vi "Clusters.vi"() -> ()   [LabVIEW 2020]
panel:
  out "cluster 2":T1
  out "cluster":T2
  in  "Array 2":dbl[](array[knob]) scale=0.0..10.0
  out "array":bool[](array[boolean])
  in  "Cluster":T3
  out "output cluster 2":T4
  in  "Array":bool[](array[boolean])
  in  "Tank":i16(slide) scale=0.0..10.0
  in  "String":string
  in  "Horizontal Pointer Slide":dbl(slide) scale=0.0..10.0
  out "output cluster":T5
  out "RPM 2":dbl
  in  "Knob":dbl(knob) scale=0.0..10.0
  out "Stop Button":bool
  out "RPM":dbl
  out "Motor1":bool
  out "Send Data":string
  out "Termocupla":dbl
  in  "Cluster1":T5 {"RPM" scale=0.0..10.0; "Termocupla" scale=0.0..100.0}
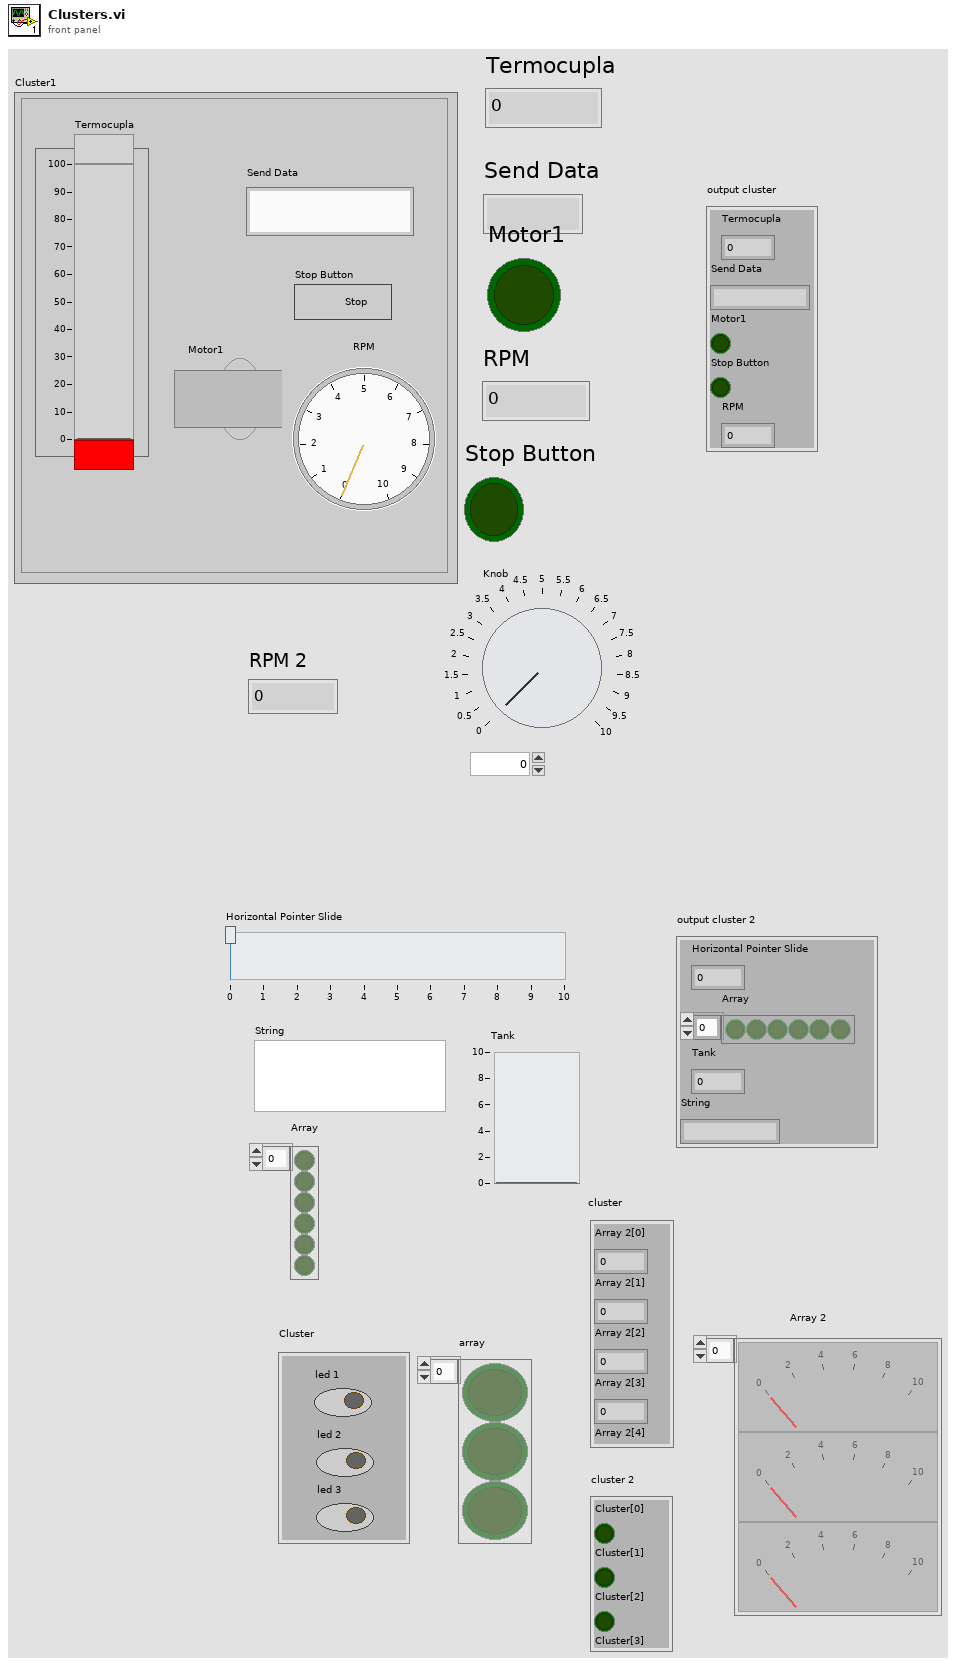
[diagram p1: front panel]
types:
  T1 = cluster{"Cluster[0]":bool, "Cluster[1]":bool, "Cluster[2]":bool, "Cluster[3]":bool, "Cluster[4]":bool, "Cluster[5]":bool, "Cluster[6]":bool, "Cluster[7]":bool, "Cluster[8]":bool}
  T2 = cluster{"Array 2[0]":dbl, "Array 2[1]":dbl, "Array 2[2]":dbl, "Array 2[3]":dbl, "Array 2[4]":dbl, "Array 2[5]":dbl, "Array 2[6]":dbl, "Array 2[7]":dbl, "Array 2[8]":dbl}
  T3 = cluster{"led 1":bool, "led 2":bool, "led 3":bool}
  T4 = cluster{"Horizontal Pointer Slide":dbl, "Array":bool[], "Tank":i16, "String":string}
  T5 = cluster{"Termocupla":dbl, "Send Data":string, "Motor1":bool, "Stop Button":bool, "RPM":dbl}
  T6 = cluster{"data_stm32":cluster{"adc":dbl[], "humedad":dbl, "status_Hardware":bool}, "data_s71200":cluster{"direccion ip":string, "puerto":i32, "termocuplas":dbl[], "sensor de nivel":dbl[]}, "node_red":cluster{"dominio":string, "puerto tcp":i32, "token":string, "api label":string, "data json":string, "formato":string, "data":dbl}, "hmi":cluster{"ktp900":string}}
  T7 = cluster{"adc":dbl[], "humedad":dbl, "status_Hardware":bool}
  T8 = cluster{"direccion ip":string, "puerto":i32, "termocuplas":dbl[], "sensor de nivel":dbl[]}
  T9 = cluster{"dominio":string, "puerto tcp":i32, "token":string, "api label":string, "data json":string, "formato":string, "data":dbl}
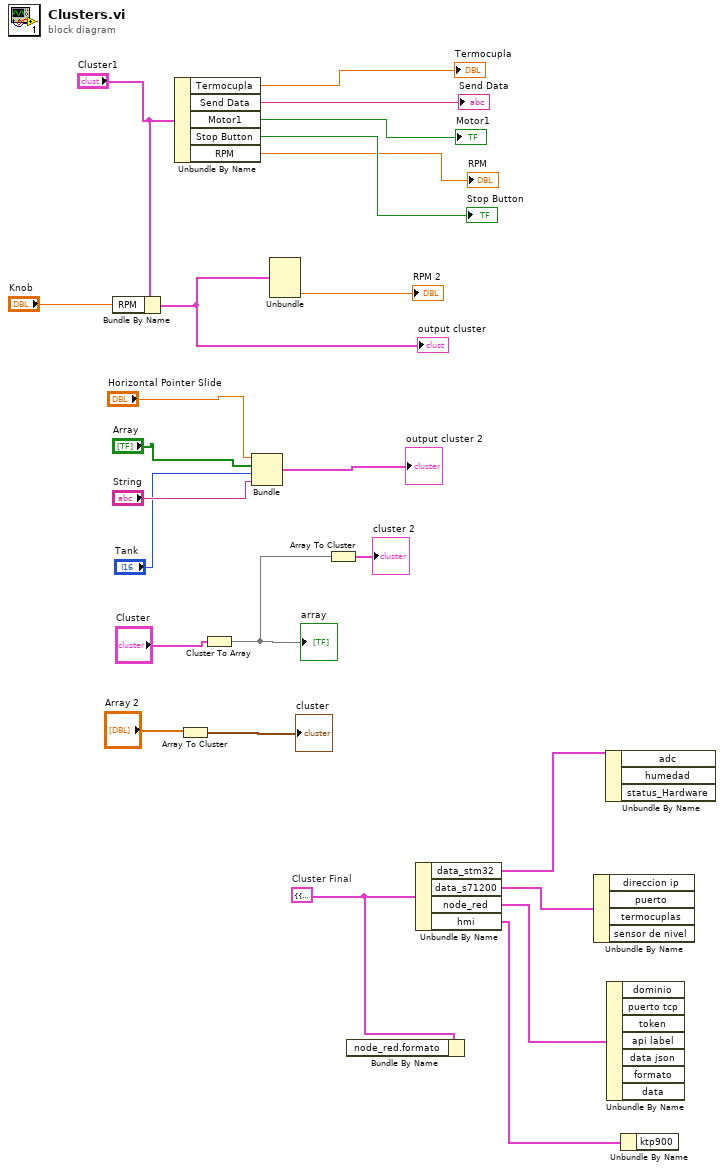
[diagram p0: block diagram]
diagram:
  w1 = T6 {"data_stm32"={"adc"=[25.0, 30.0], "humedad"=20.0, "status_Hardware"=TRUE}, "data_s71200"={"direccion ip"="192.168.1.1", "puerto"=80, "termocuplas"=[25.0, 30.0], "sensor de nivel"=[25.0, 30.0]}, "node_red"={"dominio"="nodered.com", "puerto tcp"=80, "token"="JSJan35s", "api label"="sensores", "data json"="json", "formato"="http", "data"=28.5}, "hmi"={"ktp900"="Labview 2022"}}  # Cluster Final
  n1 = Bundle By Name(cluster="Cluster1", "RPM"="Knob") -> (w17:T5)
  "output cluster" <- w17
  n2 = Unbundle By Name("Cluster1") -> ("Termocupla"=→"Termocupla":dbl, "Send Data"=→"Send Data":string, "Motor1"=→"Motor1":bool, "Stop Button"=→"Stop Button":bool, "RPM"=→"RPM":dbl)
  n3 = Array To Cluster(array="Array 2") -> (cluster=→"cluster":T2)
  n4 = Cluster To Array(cluster="Cluster") -> (array=w7:bool[])
  "array" <- w7
  n5 = Bundle("Horizontal Pointer Slide"="Horizontal Pointer Slide", "Array"="Array", "Tank"="Tank", "String"="String") -> (→"output cluster 2":T4)  [unwired: 1 in]
  n6 = Unbundle(w17) -> ("RPM"=→"RPM 2":dbl)  [unwired: 4 out]
  n7 = Array To Cluster(array=w7) -> (cluster=→"cluster 2":T1)
  n8 = Bundle By Name(cluster=w1) -> ()  [unwired: 1 in, 1 out]
  n9 = Unbundle By Name(w1) -> ("data_stm32"=w5:T7, "data_s71200"=w4:T8, "node_red"=w3:T9, "hmi"=w2:cluster{"ktp900":string})
  n10 = Unbundle By Name(w4) -> ()  [unwired: 4 out]
  n11 = Unbundle By Name(w5) -> ()  [unwired: 3 out]
  n12 = Unbundle By Name(w3) -> ()  [unwired: 7 out]
  n13 = Unbundle By Name(w2) -> ()  [unwired: 1 out]
